vi "Init All System Mappings Tab.vi"(8 "error in (no error)":errorcluster, 11 "Loop Data in":T1) -> (0 "error out":errorcluster)   [LabVIEW 2016, in "System Mapping Tool.lvlib"]
uses:
  System Mapping Tool.lvlib
  TypeDefs/Loop Data.ctl
  TypeDefs/UI Refs.ctl
  NationalInstruments.VeriStand.SystemDefinitionAPI
  NationalInstruments.VeriStand.SystemStorageUI
  <vilib>/Utility/miscctls.llb/LVRowAndColumnTypeDef.ctl
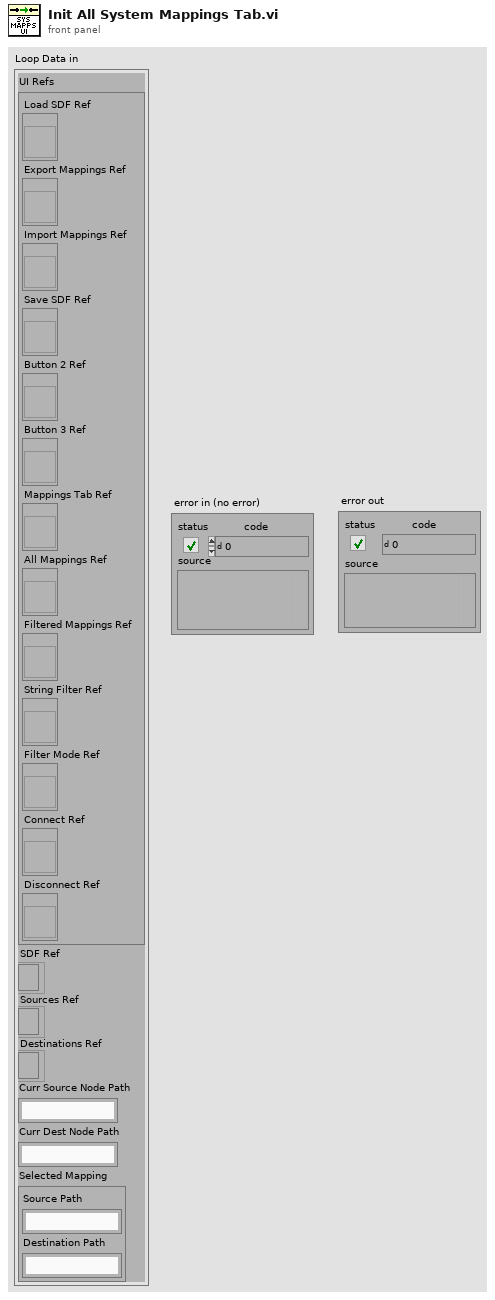
[diagram p1: front panel]
types:
  T1 = typedef "System Mapping Tool.lvlib/Loop Data.ctl" = cluster{"UI Refs":T2, "SDF Ref":refnum<k24>, "Sources Ref":refnum<k24>, "Destinations Ref":refnum<k24>, "Curr Source Node Path":string, "Curr Dest Node Path":string, "Selected Mapping":cluster{"Source Path":string, "Destination Path":string}}
  T2 = typedef "System Mapping Tool.lvlib/UI Refs.ctl" = cluster{"Load SDF Ref":refnum<vi>, "Export Mappings Ref":refnum<vi>, "Import Mappings Ref":refnum<vi>, "Save SDF Ref":refnum<vi>, "Button 2 Ref":refnum<vi>, "Button 3 Ref":refnum<vi>, "Mappings Tab Ref":refnum<vi>, "All Mappings Ref":refnum<vi>, "Filtered Mappings Ref":refnum<vi>, "String Filter Ref":refnum<vi>, "Filter Mode Ref":refnum<vi>, "Connect Ref":refnum<vi>, "Disconnect Ref":refnum<vi>}
  T3 = typedef "LVRowAndColumnTypeDef.ctl" = cluster{"Row":i32, "Column":i32}
  T4 = enum32{"All System Mappings", "Filtered Mappings by Node"}
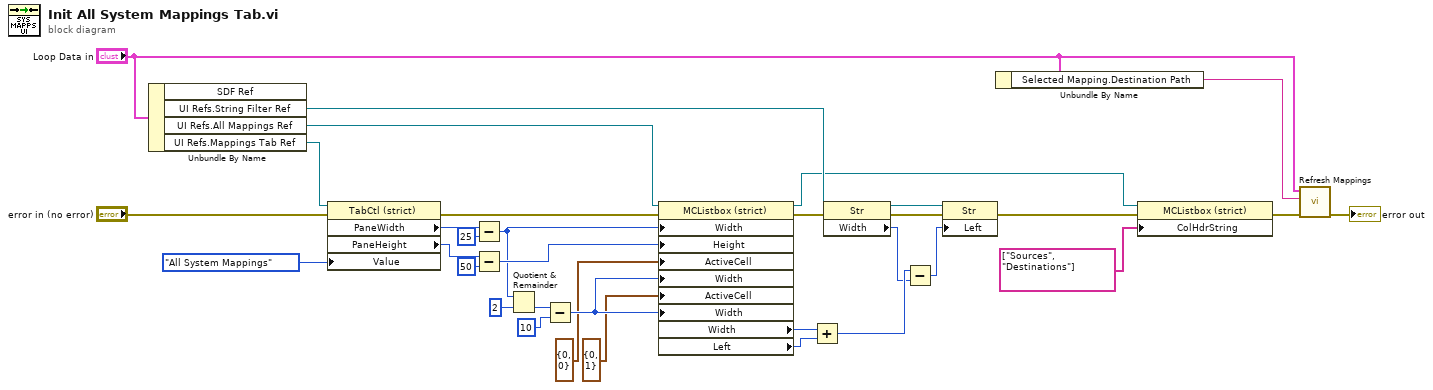
[diagram p0: block diagram]
diagram:
  n1 = Unbundle By Name("Loop Data in") -> ("UI Refs.String Filter Ref"=w14:refnum<vi>, "UI Refs.All Mappings Ref"=w20:refnum<vi>, "UI Refs.Mappings Tab Ref"=w21:refnum<vi>)  [unwired: 1 out]
  n2 = property class="TabCtl (strict)"(reference=w21, error in="error in (no error)", "Value"=T4."All System Mappings") -> (error out=w33:errorcluster, "PaneWidth"=w27:u32, "PaneHeight"=w24:u32)  [unwired: 1 out]
  n3 = Subtract(x=w27, y=u32 25) -> (x-y=w22:u32)
  n4 = Subtract(x=w24, y=u32 50) -> (x-y=w23:u32)
  n5 = Quotient & Remainder(x=w22, y=u32 2) -> (floor(x/y)=w31:u32)  [unwired: 1 out]
  n6 = Subtract(x=w31, y=u32 10) -> (x-y=w29:u32)
  n7 = property class="MCListbox (strict)"(reference=w20, error in=w33, "Width"=w22, "Height"=w23, "ActiveCell"=T3 {"Row"=0, "Column"=0} ("Active Cell:Active Cell"), "Width"=w29, "ActiveCell"=T3 {"Row"=0, "Column"=1} ("Active Cell:Active Cell"), "Width"=w29) -> (reference out=w7:refnum<vi>, error out=w12:errorcluster, "Width"=w16:u32, "Left"=w17:i32)
  n8 = Add(x=w16, y=w17) -> (x+y=w11:u32)
  n9 = property class="Str"(reference=w14, error in=w12) -> (reference out=w13:refnum<vi>, error out=w15:errorcluster, "Width"=w10:u32)
  n10 = Subtract(x=w11, y=w10) -> (x-y=w9:u32)
  n11 = property class="Str"(reference=w13, error in=w15, "Left"=w9) -> (error out=w5:errorcluster)  [unwired: 1 out]
  n12 = Unbundle By Name("Loop Data in") -> ("Selected Mapping.Destination Path"=w1:string)
  n13 = property class="MCListbox (strict)"(reference=w7, error in=w5, "ColHdrString"=string[] ["Sources", "Destinations"] ("Row Header Strings[]")) -> (error out=w8:errorcluster)  [unwired: 1 out]
  n14 = call "Refresh Mappings.vi"("error in (no error)"=w8, "Destination to Highlight"=w1, "Loop Data"="Loop Data in") -> ("error out"=→"error out":errorcluster)  [unwired: 8 in]
